vi "Transform.vi"(8 "error in (no error)":errorcluster caption="entrée d'erreur (pas d'erreur)", 10 "Image":cluster{"Array":i32[][]}[](array[cluster]), 11 "PatchExtractor.lvclass":refnum<class "PatchExtractor.lvclass">) -> (0 "error out":errorcluster caption="sortie d'erreur", 2 "Data":T1, 3 "PatchExtractor.lvclass":refnum<class "PatchExtractor.lvclass">)   [LabVIEW 2020, in "PatchExtractor.lvclass"]
doc: "Transforms the image samples in X into a matrix of patch data.\n\nReturns : \n\n- patches : array of shape (n_patches, patch_height, patch_width) or (n_patches, patch_height, patch_width, n_channels)\nThe collection of patches extracted from the images, where n_patches is either n_samples * max_patches or the total number of patches that can be extracted."
uses:
  PatchExtractor.lvclass
  PatchExtractor.lvclass/PatchExtractor.ctl
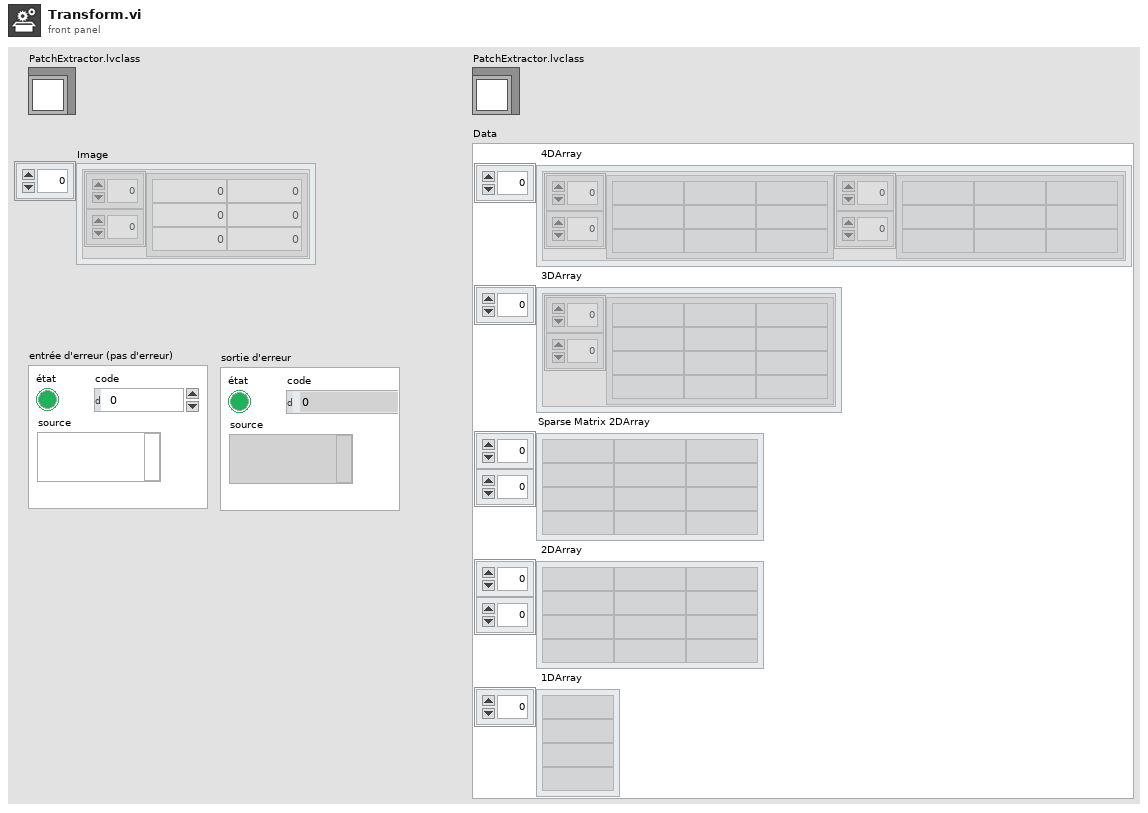
[diagram p1: front panel]
types:
  T1 = cluster{" 4DArray":cluster{"1":string[][], "2":string[][]}[], " 3DArray":cluster{"Tableau":string[][]}[], "Sparse Matrix 2DArray":string[][], " 2DArray":string[][], " 1DArray":string[]}
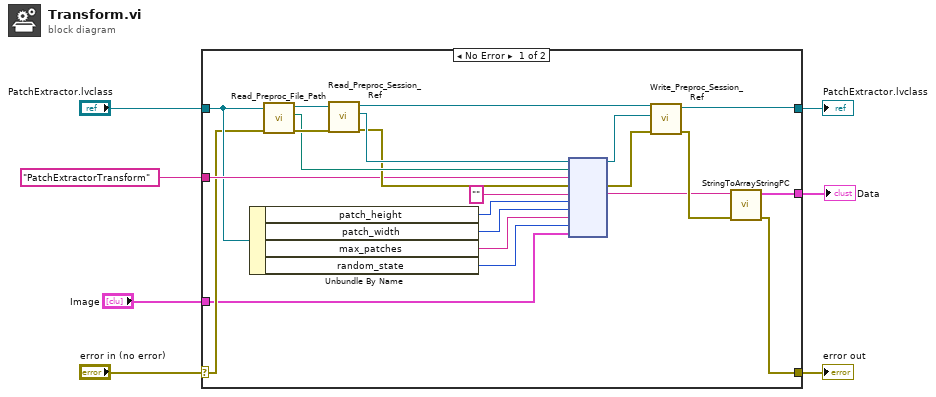
[diagram p0: block diagram]
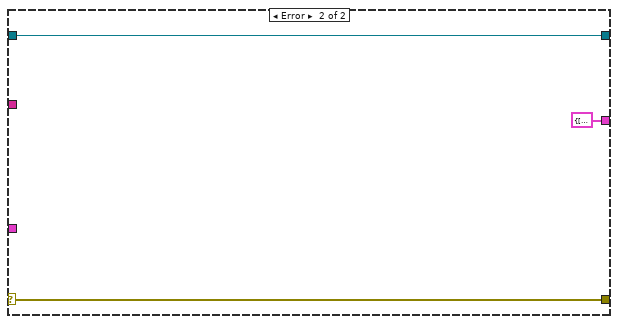
[diagram p2: hidden frame]
diagram:
  n1 = case shown="No Error" "error in (no error)" {
    selector: "error in (no error)" -> [w14 w32]
    tunnel: [w9 w32] -> w6
    tunnel: [w13 w31] -> w4
    tunnel: "PatchExtractor.lvclass" -> [w19 w31]
    tunnel: "PatchExtractorTransform" ("Fonction") -> [w20 _]
    tunnel: "Image" -> [w8 _]
    tunnel: [w10 T1 {" 4DArray"=[], " 3DArray"=[], "Sparse Matrix 2DArray"=[], " 2DArray"=[], " 1DArray"=[]} ("Data")] -> w1
    frame No Error {
      n2 = Unbundle By Name(w19) -> ("patch_height"=w18:i32, "patch_width"=w17:i32, "max_patches"=w16:string, "random_state"=w15:i32)
      n3 = call-dynamic "Read_Preproc_File_Path.vi"("error in (no error)"=w14, "Python in"=w19) -> ("error out"=w28:errorcluster, "File_Path"=w27:path, "Python out"=w29:refnum<class "PatchExtractor.lvclass">)  [unwired: 7 in]
      n4 = call-dynamic "Read_Preproc_Session_Ref.vi"("error in (no error)"=w28, "Python in"=w29) -> ("error out"=w25:errorcluster, "Session_ref"=w26:refnum<k35>, "Python out"=w24:refnum<class "PatchExtractor.lvclass">)  [unwired: 7 in]
      n5 = node(w26, w27, w20, w25, "", w18, w17, w16, w15, w8) -> (w22:refnum<k35>, w23:errorcluster, w11:string)  [unwired: 5 in, 2 out]
      n6 = call-dynamic "Write_Preproc_Session_Ref.vi"("error in (no error)"=w23, "Session_ref"=w22, "Python in"=w24) -> ("error out"=w12:errorcluster, "Python out"=w13:refnum<class "PatchExtractor.lvclass">)  [unwired: 7 in]
      n7 = call "StringToArrayStringPC.vi"("sortie d'erreur"=w12, "Return value"=w11) -> ("sortie d'erreur"=w9:errorcluster, "Data"=w10:T1)  [unwired: 8 in]
    }
    frame Error {
    }
  }
  "error out" <- w6
  "PatchExtractor.lvclass" <- w4
  "Data" <- w1
